vi "From WAMP Message.vi"(8 "error in (no error)":errorcluster, 11 "JSONMessage":refnum<class "JSONMessage.lvclass">) -> (0 "error out":errorcluster, 3 "IJsonMessageHandler":refnum<class "IJsonMessageHandler.lvclass">)   [LabVIEW 2020]
uses:
  IJsonMessageHandler.lvclass/IJsonMessageHandler.ctl
  IJsonMessageHandler.lvclass
  C:/local/wamplv/Private/Requests/MessageReceivedHandlers/IReceivedMessageHandler/IReceivedMessageHandler.lvclass
  C:/local/wamplv/Private/Requests/IInternalRequest.lvclass
  C:/local/wamplv/Private/Requests/MessageReceivedHandlers/IJsonMessageHandler/IJsonMessageHandler.lvclass
  SerialisedMessages/JSONMessage/JSONMessage.lvclass
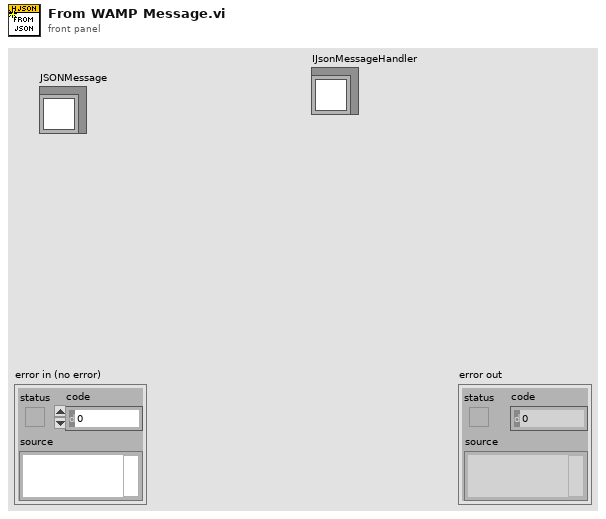
[diagram p1: front panel]
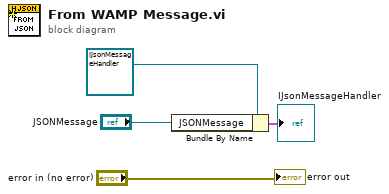
[diagram p0: block diagram]
diagram:
  n1 = Bundle By Name(cluster=refnum<class "IJsonMessageHandler.lvclass"> refnum ("wamplv.lvlib:IJsonMessageHandler.lvclass"), "JSONMessage"="JSONMessage") -> (→"IJsonMessageHandler":cluster{})
  "error out" <- "error in (no error)"
